vi "createPanel.vi"(8 "error in (no error)":errorcluster, 10 "Pane VI":string="GameOption.vi", 11 "PanelFactory in":refnum<class "PanelFactory.lvclass">) -> (0 "error out":errorcluster, 2 "Panel out":refnum<class "Panel.lvclass">)   [LabVIEW 2018, in "PanelFactory.lvclass"]
uses:
  PanelFactory.lvclass
  Panel/Panel.lvclass
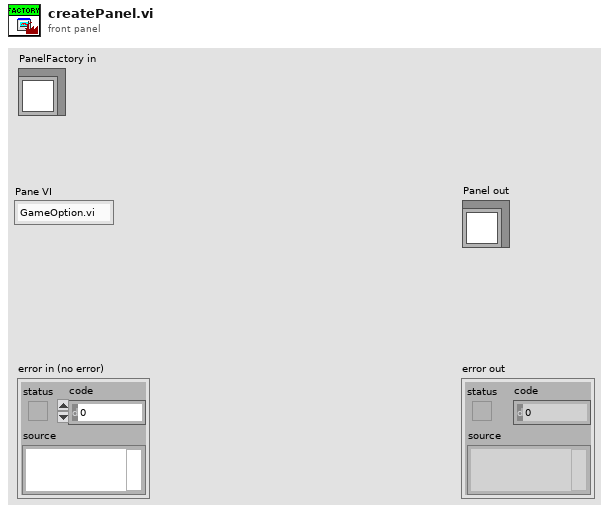
[diagram p1: front panel]
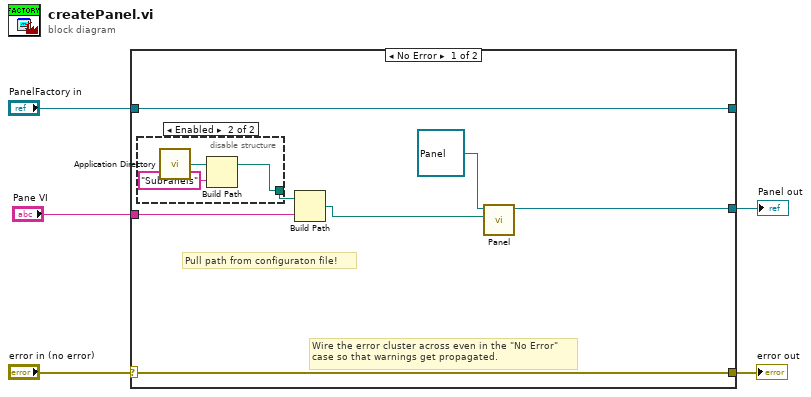
[diagram p0: block diagram]
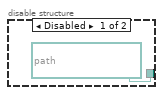
[diagram p2: hidden frame]
diagram:
  n1 = case shown="No Error" "error in (no error)" {
    selector: "error in (no error)" -> [w11 w18]
    tunnel: [w11 w18] -> w4
    tunnel: [w12 w17] -> _
    tunnel: "PanelFactory in" -> [w12 w17]
    tunnel: [w8 _] -> w2
    tunnel: "Pane VI" -> [w6 _]
    frame No Error {
      # "Pull path from configuraton file!"
      # "Wire the error cluster across even in the \"No Error\"\ncase so that warnings get propagated."
      n2 = disable-structure shown="Enabled" {
        disable-tunnel: [path "C:/Users/fflores/Documents/Interns Projects/Jogo da Velha - Lígia/Support VIs" w15] -> w9
        frame Disabled {
        }
        frame Enabled {
          n3 = call <vilib>:"Application Directory.vi"() -> ("Application Directory"=w16:path)
          n4 = Build Path(base path=w16, name or relative path="SubPanels") -> (appended path=w15:path)
        }
      }
      n5 = Build Path(base path=w9, name or relative path=w6) -> (appended path=w7:path)
      n6 = call "Panel.vi"("VI Panel Path"=w7, "Panel in"=refnum<class "Panel.lvclass"> refnum ("Panel.lvclass")) -> ("Panel out"=w8:refnum<class "Panel.lvclass">)  [unwired: 8 in, 1 out]
    }
    frame Error {
    }
  }
  "error out" <- w4
  "Panel out" <- w2
